vi "FTW-CodeGen-FindGObject.vi"(0 "GObject to Traverse":refnum<vi>, 5 "Class Type Reference":variant, 7 "Label Override":string, 11 "error in":errorcluster) -> (4 "GObject to Traverse out":refnum<vi>, 6 "GObject":refnum<vi>, 15 "error out":errorcluster)   [LabVIEW 2015]
panel:
  # "Inputs"
  # "Outputs"
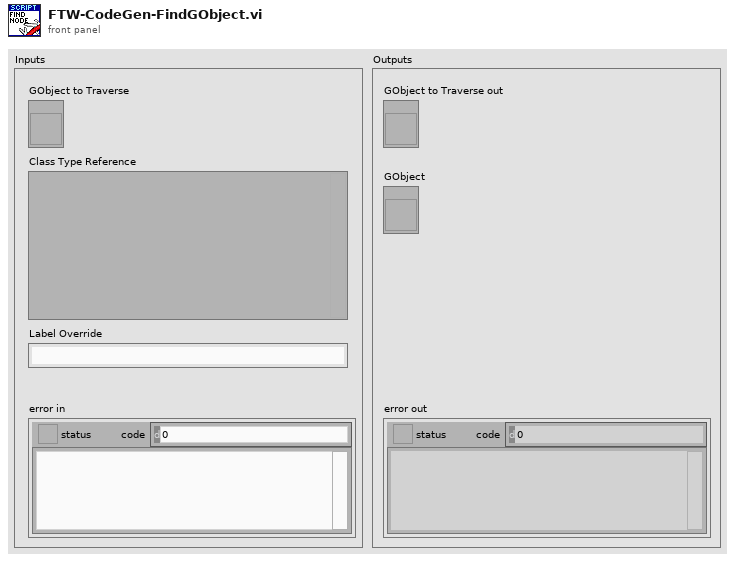
[diagram p1: front panel]
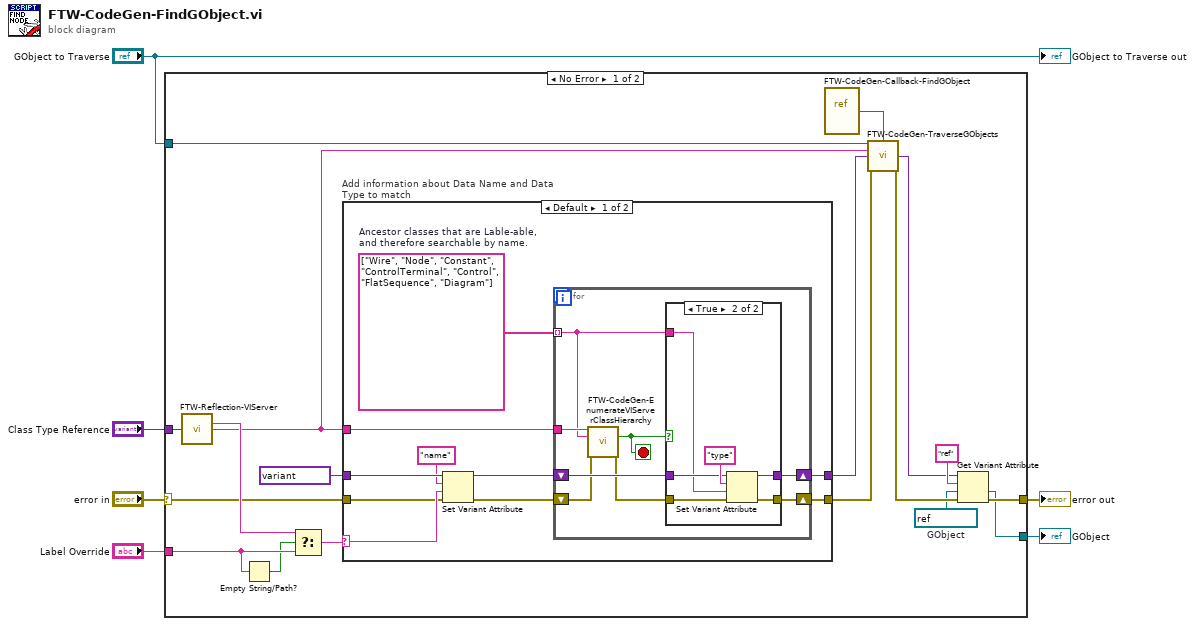
[diagram p0: block diagram]
diagram:
  n1 = case shown="No Error" "error in" {
    selector: "error in" -> [w8 w53]
    tunnel: [w10 _] -> w1
    tunnel: [w11 w53] -> w2
    tunnel: "Class Type Reference" -> [w21 _]
    tunnel: "GObject to Traverse" -> [w23 _]
    tunnel: "Label Override" -> [w17 _]
    frame No Error {
      w13 = refnum<vi> refnum  # GObject
      n2 = call "FTW-Reflection-VIServer.vi"("VI Server Reference"=w21) -> ("Data Name"=w16:string, "Class Name"=w7:string)  [unwired: 11 in, 2 out]
      n3 = Empty String/Path?(string/path=w17) -> (empty?=w15:bool)
      n4 = Select(t=w16, s=w15, f=w17) -> (s? t:f=w9:string)
      n5 = case "Add information about Data Name and Data Type to match" shown="Default" w9 {
        selector: w9 -> [w32 _]
        tunnel: variant ("variant") -> [w34 w52]
        tunnel: [w25 w51] -> w20
        tunnel: [w26 w52] -> w18
        tunnel: w8 -> [w31 w51]
        tunnel: w7 -> [w30 _]
        frame Default {
          w29 = string[] ["Wire", "Node", "Constant", "ControlTerminal", "Control", "FlatSequence", "Diagram"]  # Ancestor classes that are Lable-able, and therefore searchable by name.
          n6 = Set Variant Attribute(Variant=w34, name="name", value=w32, error in=w31) -> (Variant out=w28:variant, error out=w27:errorcluster)  [unwired: 1 out]
          n7 = for {
            tunnel: w30 -> [w42]
            tunnel: w29 -> [w36] mode=indexing
            shift-right: [w40] -> w26
            shift-left: w28 -> [w41]
            shift-right: [w39] -> w25
            shift-left: w27 -> [w38]
            stop <- w35 stop-if-true
            n8 = call "FTW-CodeGen-EnumerateVIServerClassHierarchy.vi"("Class"=w42, "Ancestor"=w36, "error in"=w38) -> ("Is Descendent?"=w35:bool, "error out"=w37:errorcluster)  [unwired: 11 in]
            n9 = case shown="True" w35 {
              tunnel: w41 -> [w44 w49]
              tunnel: [w44 w48] -> w40
              tunnel: w37 -> [w43 w47]
              tunnel: [w43 w46] -> w39
              tunnel: w36 -> [_ w45]
              frame False {
              }
              frame True {
                n10 = Set Variant Attribute(Variant=w49, name="type", value=w45, error in=w47) -> (Variant out=w48:variant, error out=w46:errorcluster)  [unwired: 1 out]
              }
            }
          }
        }
        frame "" {
        }
      }
      n11 = vi-ref "FTW-CodeGen-Callback-FindGObject.vi"() -> (w24:refnum<vi>)
      n12 = call "FTW-CodeGen-TraverseGObjects.vi"("GObject to Traverse"=w23, "GObject Filter Callback"=w24, "Class Name"=w7, "Initial Context"=w18, "error in"=w20) -> ("Final Context"=w12:variant, "error out"=w19:errorcluster)  [unwired: 9 in]
      n13 = Get Variant Attribute(Variant=w12, name="ref", default value (empty Variant)=w13, error in=w19) -> (value=w10:refnum<vi>, error out=w11:errorcluster)  [unwired: 2 out]
    }
    frame Error {
    }
  }
  "error out" <- w2
  "GObject" <- w1
  "GObject to Traverse out" <- "GObject to Traverse"
